vi "Convert String To String.vi"(8 "error in (no error)":errorcluster, 9 "Value":string, 11 "Str Refnum":refnum<vi>) -> (0 "error out":errorcluster)   [LabVIEW 2013]
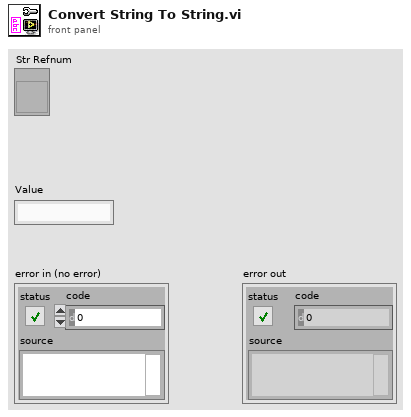
[diagram p1: front panel]
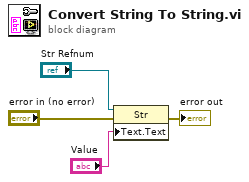
[diagram p0: block diagram]
diagram:
  n1 = property class="Str"(reference="Str Refnum", error in="error in (no error)", "Text.Text"="Value") -> (error out=→"error out":errorcluster)  [unwired: 1 out]
